vi "Read_password_example.vi"() -> ()   [LabVIEW 2016]
uses:
  <vilib>/Utility/miscctls.llb/LVPointTypeDef.ctl
  Access/Access Lib.lvlib
panel:
  in  "数据库路径":path
  in  "读取秘钥":bool
  in  "去除秘钥":bool
  in  "取消按钮":bool
  in  "password":string
  # "数据库秘钥"
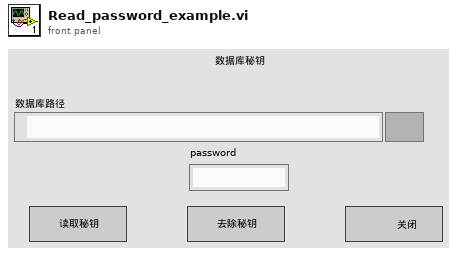
[diagram p1: front panel]
types:
  T1 = typedef "LVPointTypeDef.ctl" = cluster{"Horizontal":i16, "Vertical":i16}
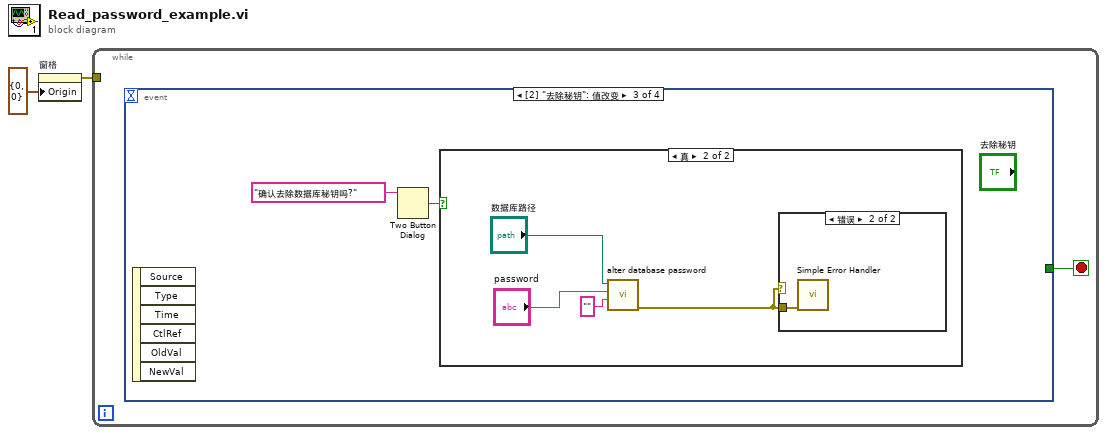
[diagram p0: block diagram]
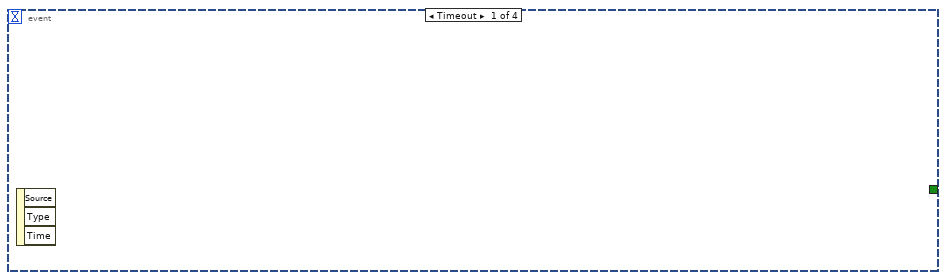
[diagram p2: hidden frame]
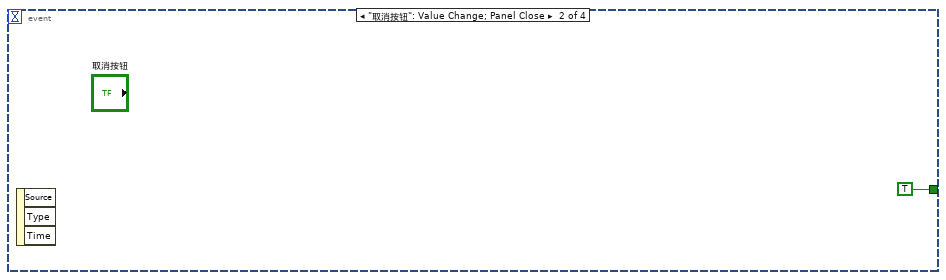
[diagram p3: hidden frame]
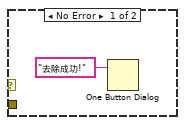
[diagram p5: hidden frame]
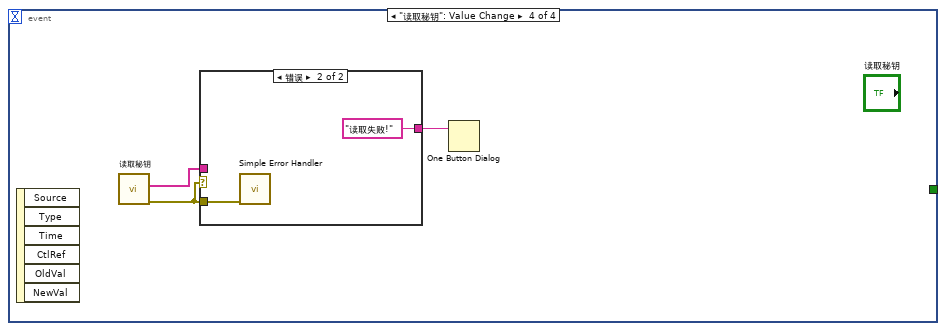
[diagram p6: hidden frame]
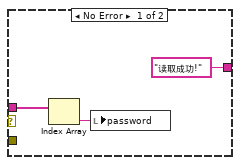
[diagram p7: hidden frame]
diagram:
  n1 = property on="窗格" class="Pane"("Origin"=T1 {"Horizontal"=0, "Vertical"=0} ("原点")) -> (error out=w1:errorcluster)  [unwired: 2 in, 1 out]
  n2 = while {
    tunnel: w1 -> [_]
    stop <- w3 stop-if-true
    n3 = event shown="[2] \"去除秘钥\": 值改变" {
      selector: _ -> [_ _ _ _]
      dyn-events: _ -> [_ _ _ _]
      timeout: _ -> [_ _ _ _]
      tunnel: [_ TRUE _ _] -> w3
      event Timeout {
        n4 = event-data() -> ()  [unwired: 1 in, 3 out]
      }
      event "取消按钮": Value Change; Panel Close {
        n5 = event-data() -> ()  [unwired: 1 in, 3 out]
      }
      event "去除秘钥": Value Change {
        n6 = event-data() -> ()  [unwired: 1 in, 6 out]
        n7 = Two Button Dialog(message="确认去除数据库秘钥吗?" ("消息")) -> (T button?=w5:bool)  [unwired: 2 in]
        n8 = case shown="真" w5 {
          frame False {
          }
          frame True {
            n9 = call "alter database password.vi"("NewPWd"="", "OpenPwd"="password", "路径"="数据库路径") -> ("错误输出"=w8:errorcluster)  [unwired: 8 in]
            n10 = case shown="错误" w8 {
              tunnel: w8 -> [_ w12]
              frame No Error {
                n11 = One Button Dialog(message="去除成功!" ("消息")) -> ()  [unwired: 1 in, 1 out]
              }
              frame Error {
                n12 = call <vilib>:"Simple Error Handler.vi"("error in (no error)"=w12) -> ()  [unwired: 4 in, 5 out]
              }
            }
          }
        }
      }
      event "读取秘钥": Value Change {
        n13 = event-data() -> ()  [unwired: 1 in, 6 out]
        n14 = call "读取秘钥.vi"() -> ("error out"=w13:errorcluster, "值"=w15:string[])  [unwired: 9 in, 1 out]
        n15 = case shown="错误" w13 {
          tunnel: w15 -> [w18 _]
          tunnel: ["读取成功!" ("消息") "读取失败!" ("消息")] -> w14
          tunnel: w13 -> [_ w19]
          frame No Error {
            n16 = Index Array(array=w18) -> (element=w17:string)  [unwired: 1 in]
            n17 = local write "password"(w17) -> ()
          }
          frame Error {
            n18 = call <vilib>:"Simple Error Handler.vi"("error in (no error)"=w19) -> ()  [unwired: 4 in, 5 out]
          }
        }
        n19 = One Button Dialog(message=w14) -> ()  [unwired: 1 in, 1 out]
      }
    }
  }
